vi "Teleop.vi"(10 "Match Info":T1={"Autonomous Elapsed Seconds"=0.0, "TeleOp Elapsed Seconds"=0.0, "Disabled Elapsed Seconds"=0.0, "Visited Autonomous"=FALSE, "Visited TeleOp"=FALSE, "Visited Disabled"=FALSE, "Autonomous Settings"={"Autonomous Style"=enum."Independent", "VI Refnum"=refnum}}, 11 "Call Context":T2) -> ()   [LabVIEW 2019]
doc: "This VI is called for each enabled TeleOp packet received from the DS. It is typically used to read from joysticks and other inputs and update I/O or setpoints for timed control loops. It should complete and return within 20 milliseconds or risk missing DS packets."
uses:
  <vilib>/Rock Robotics/WPI/DriverStation/WPI_DriverStationDerivedRobotMode.ctl
  <vilib>/Rock Robotics/WPI/DriverStation/WPI_DriverStationMatch Info.ctl
  <vilib>/Rock Robotics/WPI/Utilities/WPI_GetSetVariantRefNum.vi
  <vilib>/Rock Robotics/Network Tables/NT Write Boolean Array.vi
  <vilib>/Rock Robotics/Network Tables/NT Write Numeric Array.vi
  <vilib>/Rock Robotics/WPI/DriverStation/WPI_DriverStationRobotMode2.ctl
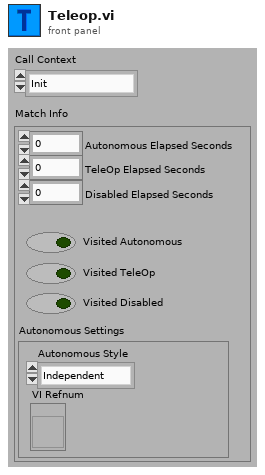
[diagram p1: front panel]
types:
  T1 = typedef "WPI_DriverStationMatch Info.ctl" = cluster{"Autonomous Elapsed Seconds":dbl, "TeleOp Elapsed Seconds":dbl, "Disabled Elapsed Seconds":dbl, "Visited Autonomous":bool, "Visited TeleOp":bool, "Visited Disabled":bool, "Autonomous Settings":cluster{"Autonomous Style":enum16{"Iterative", "Independent"}, "VI Refnum":refnum<vi>}}
  T2 = typedef "WPI_DriverStationDerivedRobotMode.ctl" = enum16{"Init", "Execute", "Stop"}
  T3 = typedef "WPI_JoystickDevRef.ctl" = cluster{"Device":T4}
  T4 = typedef "WPI_JoystickDeviceEnum.ctl" = enum16{"USB 0", "USB 1", "USB 2", "USB 3", "USB 4", "USB 5"}
  T5 = typedef "WPI_DriverStationRobotMode2.ctl" = enum16{"Autonomous Disabled", "Autonomous Enabled", "Teleop Disabled", "Teleop Enabled", "Disconnected", "Finish", "Test Disabled", "Test Enabled", "Emergency Stopped"}
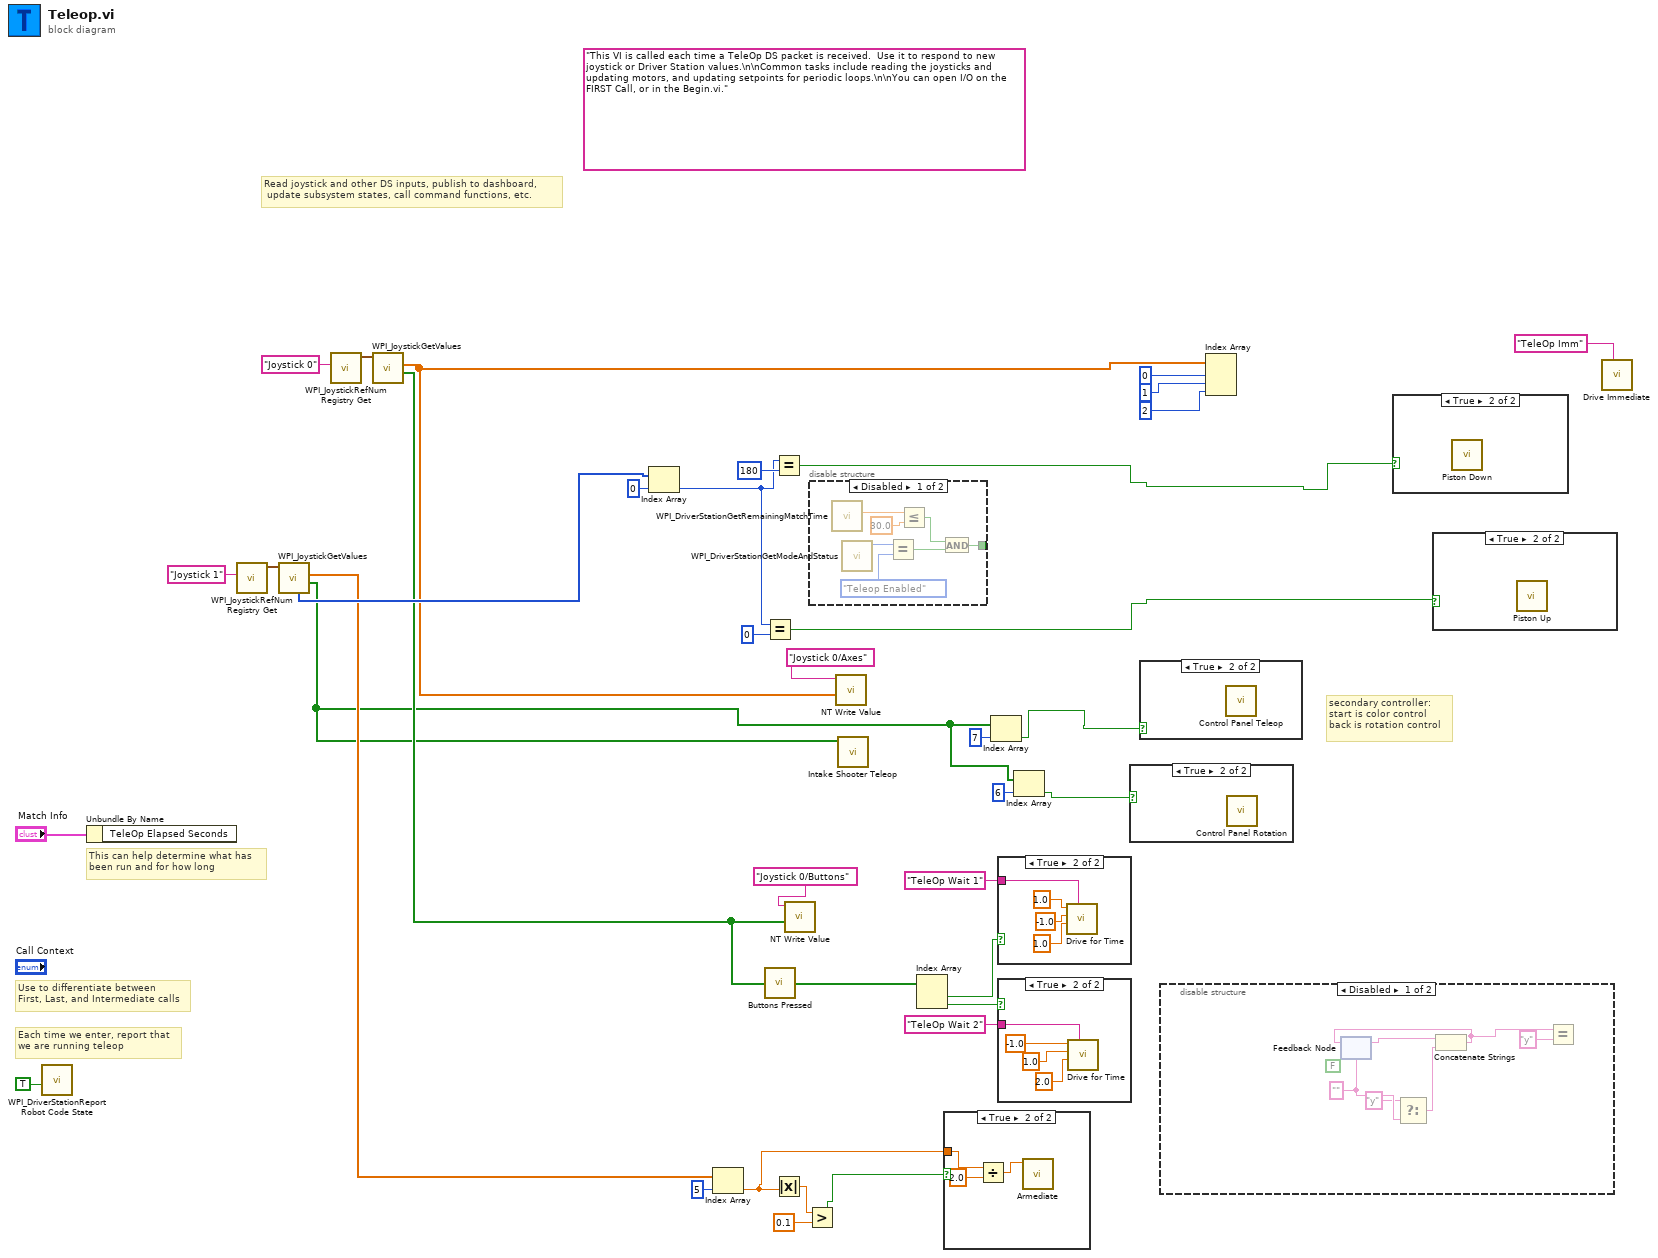
[diagram p0: block diagram]
diagram:
  (unwired) "This VI is called each time a TeleOp DS packet is received.  Use it to respond to new joystick or Driver Station values.\n\nCommon tasks include reading the joysticks and updating motors, and updating setpoints for periodic loops.\n\nYou can open I/O on the FIRST Call, or in the Begin.vi."
  # "secondary controller:\nstart is color control\nback is rotation control"
  # "Read joystick and other DS inputs, publish to dashboard,\n update subsystem states, call command functions, etc."
  # "Each time we enter, report that\nwe are running teleop"
  # "Use to differentiate between\nFirst, Last, and Intermediate calls"
  # "This can help determine what has\nbeen run and for how long"
  n1 = call <vilib>:"WPI_DriverStationReport Robot Code State.vi"("TeleOp"=TRUE ("Autonomous")) -> ()  [unwired: 10 in, 1 out]
  n2 = Unbundle By Name("Match Info") -> ()  [unwired: 1 out]
  n3 = call <vilib>:"WPI_JoystickRefNum Registry Get.vi"("refnum name"="Joystick 1") -> ("JoystickDevRef"=w24:T3)  [unwired: 1 in, 9 out]
  n4 = call <vilib>:"WPI_JoystickGetValues.vi"("JoystickDevRef"=w24) -> ("Buttons"=w6:bool[], "Axes"=w22:dbl[], "POVs"=w23:i16[])  [unwired: 6 in, 2 out]
  n5 = call <vilib>:"WPI_JoystickRefNum Registry Get.vi"("refnum name"="Joystick 0") -> ("JoystickDevRef"=w34:T3)  [unwired: 1 in, 9 out]
  n6 = call <vilib>:"WPI_JoystickGetValues.vi"("JoystickDevRef"=w34) -> ("Buttons"=w10:bool[], "Axes"=w4:dbl[])  [unwired: 6 in, 3 out]
  n7 = Index Array(array=w23, index=0) -> (element=w13:i16)
  n8 = Index Array(array=w22, index=5) -> (element=w17:dbl)
  n9 = Equal?(x=w13, y=i16 0) -> (x = y?=w12:bool)
  n10 = call "Buttons Pressed.vi"("Button Values"=w10) -> ("Button Presses"=w27:bool[])
  n11 = Equal?(x=w13, y=i16 180) -> (x = y?=w11:bool)
  n12 = Absolute Value(x=w17) -> (abs(x)=w21:dbl)
  n13 = call-poly <vilib>:"NT Write Value.vi"("Boolean Array"=w10, "Name"="Joystick 0/Buttons") -> ()  [unwired: 9 in, 1 out]
  n14 = Greater?(x=w21, y=0.1) -> (0:w19:bool)
  n15 = disable-structure shown="Disabled" {
    disable-tunnel: [w38 _] -> _
    frame Disabled {
      n16 = call <vilib>:"WPI_DriverStationGetRemainingMatchTime.vi"() -> ("Match Time(s)"=w42:sgl)  [unwired: 10 in, 1 out]
      n17 = call <vilib>:"WPI_DriverStationGetModeAndStatus.vi"() -> ("Robot Mode"=w44:T5)  [unwired: 10 in, 1 out]
      n18 = Equal?(x=w44, y=WPI_DriverStationRobotMode2."Teleop Enabled") -> (x = y?=w39:bool)
      n19 = Less Or Equal?(x=w42, y=sgl 30.0) -> (x <= y?=w40:bool)
      n20 = And(x=w40, y=w39) -> (x .and. y?=w38:bool)
    }
    frame Enabled {
    }
  }
  n21 = call-poly <vilib>:"NT Write Value.vi"("Numeric Array"=w4, "Name"="Joystick 0/Axes") -> ()  [unwired: 9 in, 1 out]
  n22 = call "Intake Shooter Teleop.vi"("Buttons"=w6) -> ()  [unwired: 11 in]
  n23 = Index Array(array=w27) -> (element #1=w31:bool, element #2=w30:bool)  [unwired: 2 in]
  n24 = case shown="True" w19 {
    tunnel: w17 -> [_ w47]
    frame False {
    }
    frame True {
      n25 = Divide(x=w47, y=2.0) -> (x/y=w45:dbl)
      n26 = call "Armediate.vi"("Setpoint"=w45) -> ()  [unwired: 10 in, 1 out]
    }
  }
  n27 = Index Array(array=w6, index=7) -> (element=w8:bool)
  n28 = case shown="True" w31 {
    tunnel: "TeleOp Wait 1" ("Description") -> [_ w50]
    frame False {
    }
    frame True {
      n29 = call "Drive for Time.vi"("Description"=w50, "Seconds"=1.0, "Right Speed"=-1.0, "Left Speed"=1.0) -> ()  [unwired: 7 in, 1 out]
    }
  }
  n30 = case shown="True" w30 {
    tunnel: "TeleOp Wait 2" ("Description") -> [_ w53]
    frame False {
    }
    frame True {
      n31 = call "Drive for Time.vi"("Description"=w53, "Seconds"=2.0, "Right Speed"=1.0, "Left Speed"=-1.0) -> ()  [unwired: 7 in, 1 out]
    }
  }
  n32 = Index Array(array=w6, index=6) -> (element=w5:bool)
  n33 = case shown="True" w5 {
    frame False {
    }
    frame True {
      n34 = call "Control Panel Rotation.vi"() -> ()  [unwired: 11 in, 1 out]
    }
  }
  n35 = case shown="True" w8 {
    frame False {
    }
    frame True {
      n36 = call "Control Panel Teleop.vi"() -> ()  [unwired: 12 in]
    }
  }
  n37 = disable-structure shown="Disabled" {
    frame Disabled {
      w57 = FALSE
      w62 = ""
      n38 = feedback #1(w62) -> (w63:string)
      n39 = Select(t="y", f=w62) -> (s=w56:bool, s? t:f=w61:string)
      n40 = Concatenate Strings(w63, w61) -> (w59:string)
      n41 = feedback-in #1(w59) -> ()
      n42 = Equal?(x=w59, y="y") -> ()  [unwired: 1 out]
    }
    frame Enabled {
    }
  }
  n43 = Index Array(array=w4, index #1=0 ("index"), index #2=1 ("index"), index #3=2 ("index")) -> ()  [unwired: 3 out]
  n44 = case shown="True" w11 {
    frame False {
    }
    frame True {
      n45 = call "Piston Down.vi"() -> ()  [unwired: 11 in, 1 out]
    }
  }
  n46 = case shown="True" w12 {
    frame False {
    }
    frame True {
      n47 = call "Piston Up.vi"() -> ()  [unwired: 11 in, 1 out]
    }
  }
  n48 = call "Drive Immediate.vi"("Description"="TeleOp Imm") -> ()  [unwired: 10 in, 1 out]
